vi "RichToFlatstreamai_signalConfig.vi"(5 "OutputClusterType":T1, 11 "InputCluster":T3) -> (3 "OutputCluster":T1)   [LabVIEW 2023, in "Generated_server.lvlib"]
uses:
  Generated_server.lvlib
  streamai_signalConfig.ctl
  streamai_SignalType.ctl
  streamai_signalConfig_Flat.ctl
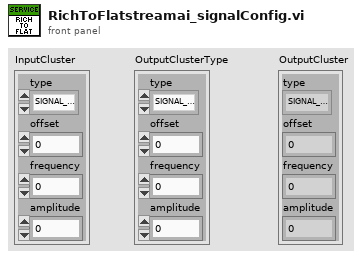
[diagram p1: front panel]
types:
  T1 = typedef "Generated_server.lvlib/streamai_signalConfig_Flat.ctl" = cluster{"type":T2, "offset":dbl, "frequency":dbl, "amplitude":dbl}
  T2 = typedef "Generated_server.lvlib/streamai_SignalType.ctl" = enum32{"SIGNAL_SINE", "SIGNAL_SQUARE"}
  T3 = typedef "Generated_server.lvlib/streamai_signalConfig.ctl" = cluster{"type":T2, "offset":dbl, "frequency":dbl, "amplitude":dbl}
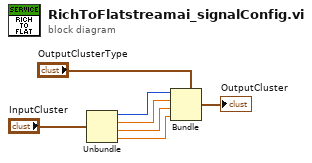
[diagram p0: block diagram]
diagram:
  n1 = Unbundle "Unbundle"("InputCluster") -> ("type"=w4:T2, "offset"=w3:dbl, "frequency"=w2:dbl, "amplitude"=w1:dbl)
  n2 = Bundle "Bundle"(cluster="OutputClusterType", "type"=w4, "offset"=w3, "frequency"=w2, "amplitude"=w1) -> (→"OutputCluster":T1)
